vi "Tree.vi"(4 "Item Name":string, 5 "Tree In":string(tree)="Item1") -> (1 "Navigate Tree:Get Path":string[](array[string]), 2 "Tree Out":string(tree)="SubItem14_1")   [LabVIEW 2010]
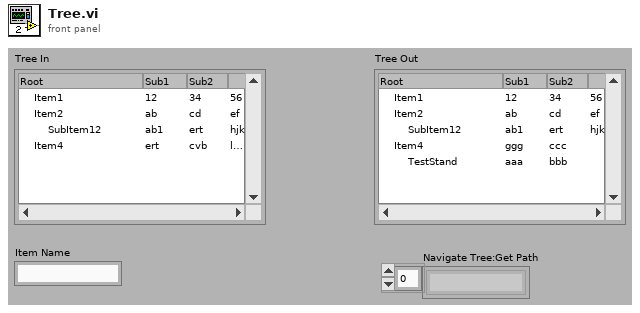
[diagram p1: front panel]
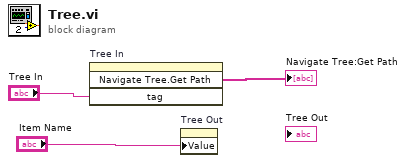
[diagram p0: block diagram]
diagram:
  n1 = invoke on="Tree In" class="Tree (strict)" method="Navigate Tree.Get Path"("tag"="Tree In") -> ("Navigate Tree:Get Path"=→"Navigate Tree:Get Path":string[])  [unwired: 3 in, 3 out]
  n2 = property on="Tree Out" class="Tree (strict)"("Value"="Item Name") -> ()  [unwired: 2 in, 2 out]
